vi "Car Wash.vi"() -> ()   [LabVIEW 2021]
uses:
  Controls/Car Wash Indicators.ctl
  Controls/Wash Options.ctl
  Controls/Enum State Machine.ctl
  <vilib>/DAQmx/read.llb/DAQmx Read (Counter U32 1Chan 1Samp).vi
  <vilib>/DAQmx/read.llb/DAQmx Read (Analog 1D Wfm NChan NSamp).vi
  <vilib>/DAQmx/write.llb/DAQmx Write (Analog 1D Wfm NChan NSamp).vi
  <vilib>/DAQmx/miscellaneous.llb/DAQmx Fill In Error Info.vi
  <vilib>/DAQmx/configure/timing.llb/DAQmx Timing (Use Waveform).vi
  <vilib>/measure/NI_MABase.lvlib
panel:
  out "Water Flow Graph":waveform(dbl)[](graph)
  in  "Duty Cycle Control(%)":dbl(slide)=5.0 min=5.0 max=95.0 step=1.0 scale=5.0..95.0 scale format="%.2g"
  out "error out":errorcluster
  in  "error in (no error)":errorcluster
  in  "Data Type":u8
  in  "Wash Options":T1
  in  "Start":bool
  out "Elapsed Time":dbl format="%0.2f"
  in  "stop":bool
  out "Wash Entry":bool
  out "Car Position Slider":u8(slide) max=3 scale=0.0..4.0
  out "CW Indicators":T2
  # "Entry Console"
  # "Car Wash Display"
  # "Car Position Simulation"
  # "Pre-Soak\nH-P Wash\nL-P Wax\nSpot Free Rinse"
  # "Underbody Wash\nBug Remover"
  # "Tire Shine\nAir Dry"
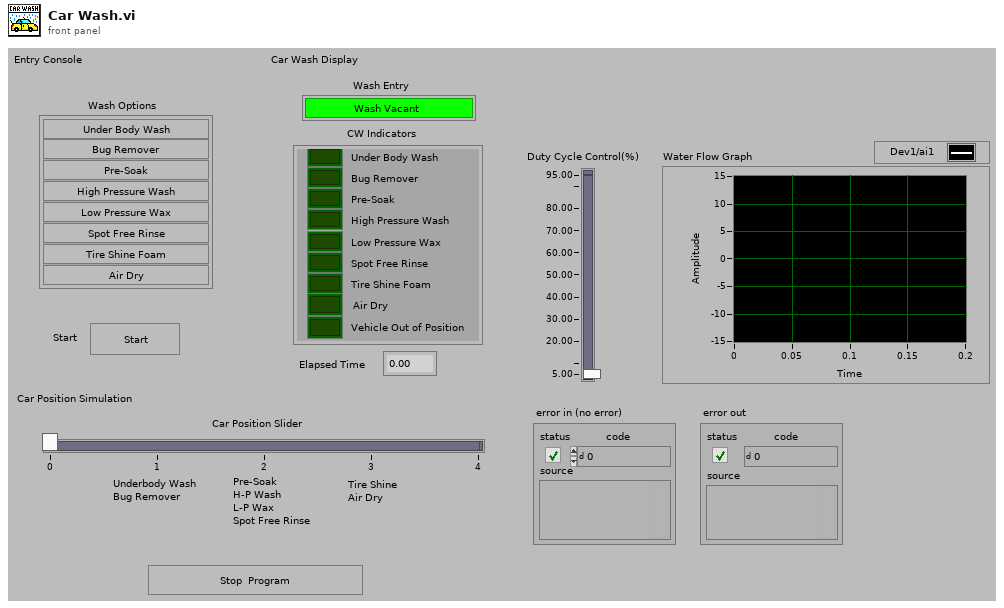
[diagram p1: front panel]
types:
  T1 = typedef "Wash Options.ctl" = cluster{"Underbody Wash":bool, "Bug Remover":bool, "Pre-Soak":bool, "High Pressure Wash":bool, "Low Pressure Wax":bool, "Spot Free Rinse":bool, "Tire Shine Foam":bool, "Air Dry":bool}
  T2 = typedef "Car Wash Indicators.ctl" = cluster{"Vehicle Out of Position":bool, "Under Body Wash":bool, "Bug Remover":bool, "Pre-Soak":bool, "High Pressure Wash":bool, "Low Pressure Wax":bool, "Spot Free Rinse":bool, "Tire Shine Foam":bool, "Air Dry":bool}
  T3 = cluster{"frequency":dbl, "amplitude":dbl, "phase":dbl, "sampling info":cluster{"Fs":dbl, "#s":dbl}}
  T4 = cluster{"maximum value":dbl, "minimum value":dbl, "physical channels":tag}
  T5 = cluster{"minimum value":dbl, "maximum value":dbl, "physical channels":tag, "rate":dbl, "sample mode":i32, "samples per channel":i32}
  T6 = cluster{"initial count":u32, "count direction":i32, "edge":i32, "counter":tag, "CI.CountEdges.Term":tag}
  T7 = typedef "Enum State Machine.ctl" = enum16{"Entry", "Under Body Wash", "Bug Remover", "Pre-Soak", "High Pressure Wash", "Low Pressure Wax", "Spot Free Rinse", "Tire Shine Foam", "Air Dry", "Exit", "Startup", "Wait for Start", "Stop"}
  T8 = cluster{"Car Wash Indicators":T2, "Wash Options":T1}
  T9 = enum8{"Enabled", "Disabled", "Disabled and Grayed Out"}
  T10 = typedef "Car Wash Data.ctl" = cluster{"Car Wash Indicators":T2, "Wash Options":T1}
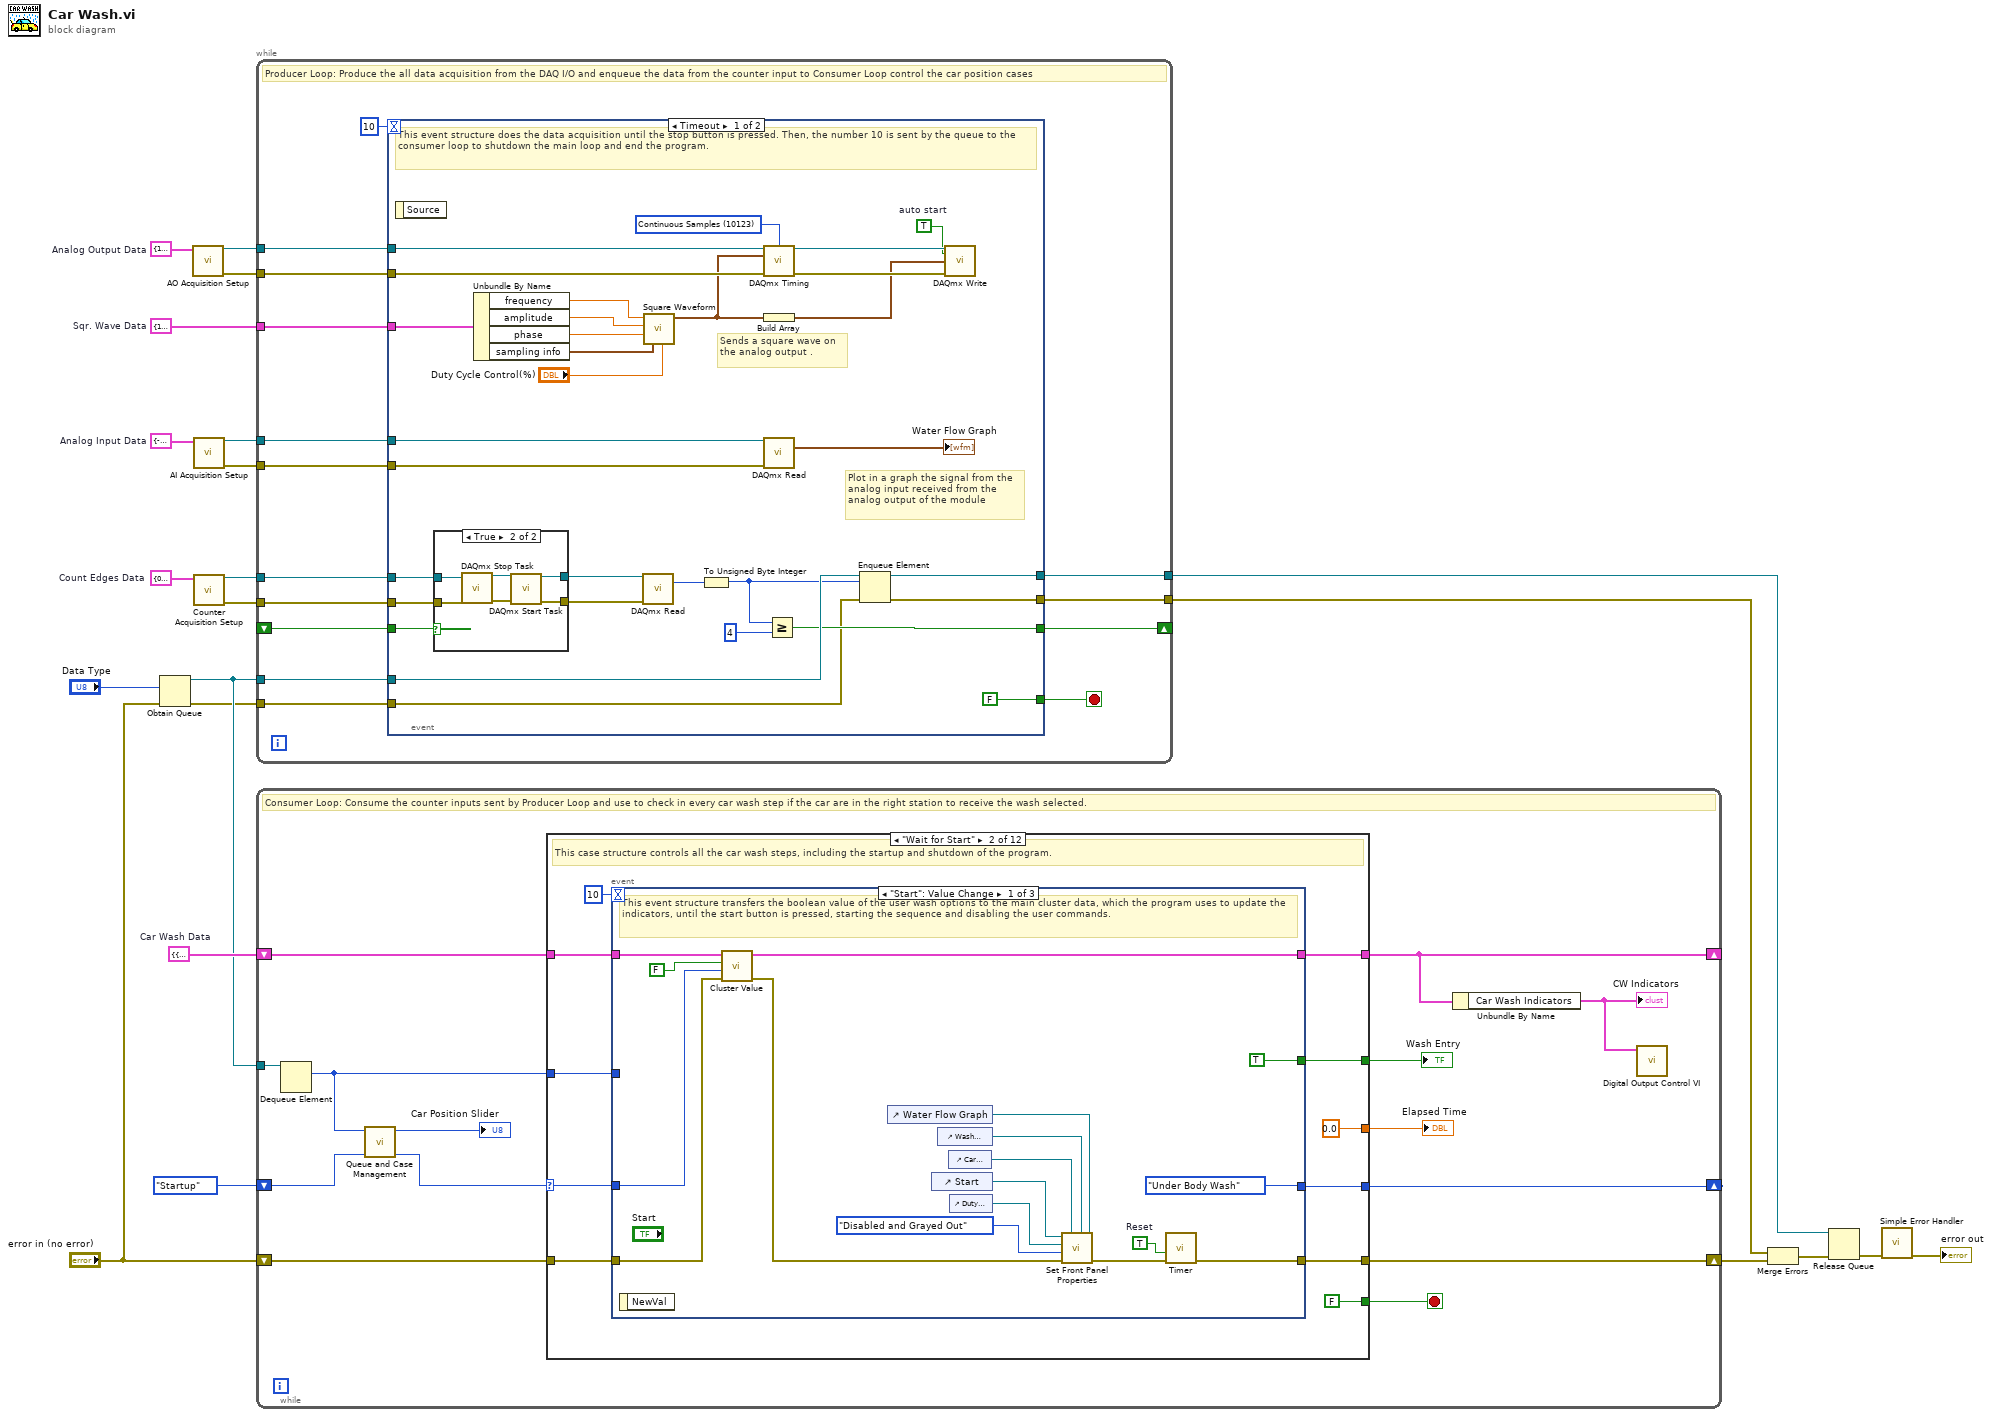
[diagram p0: block diagram]
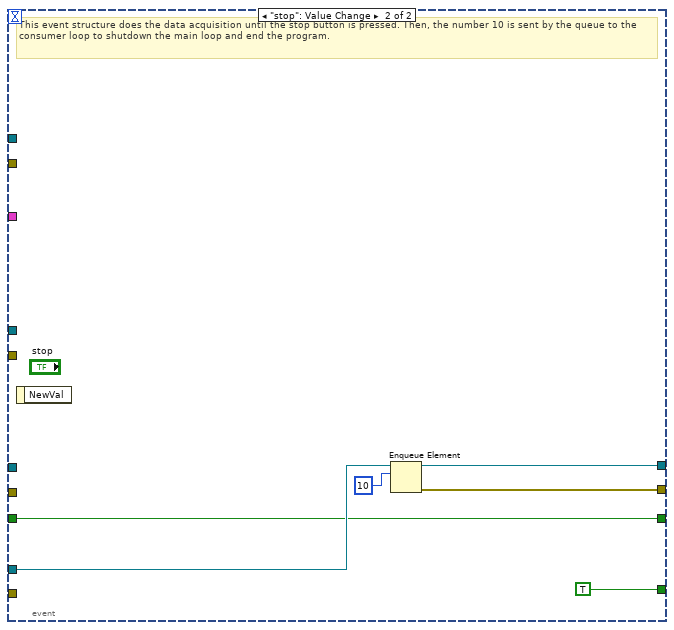
[diagram p3: hidden frame]
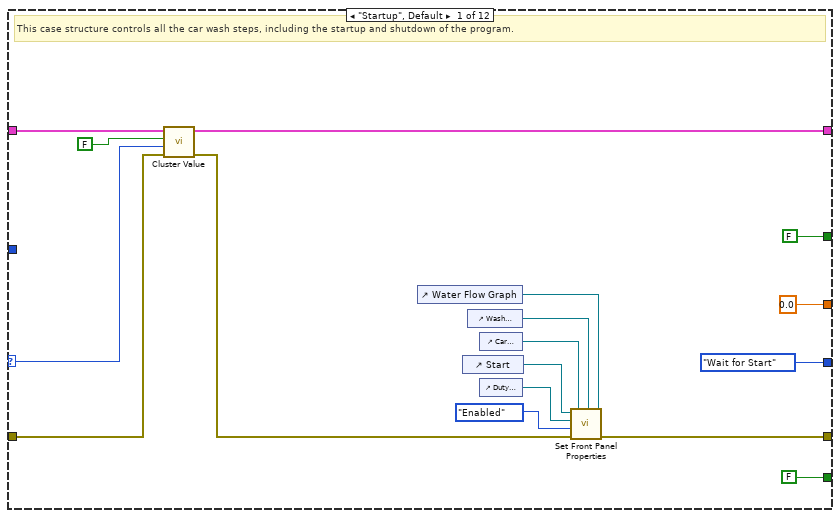
[diagram p4: hidden frame]
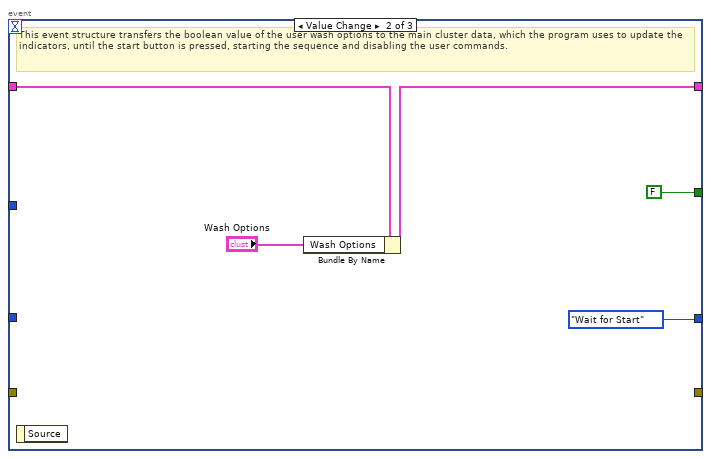
[diagram p5: hidden frame]
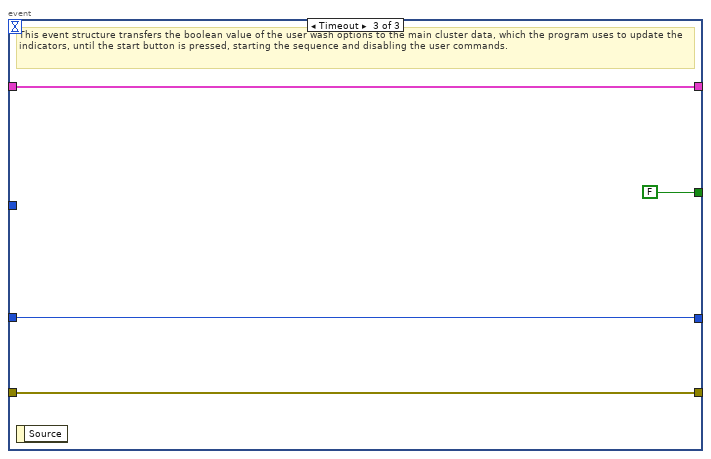
[diagram p6: hidden frame]
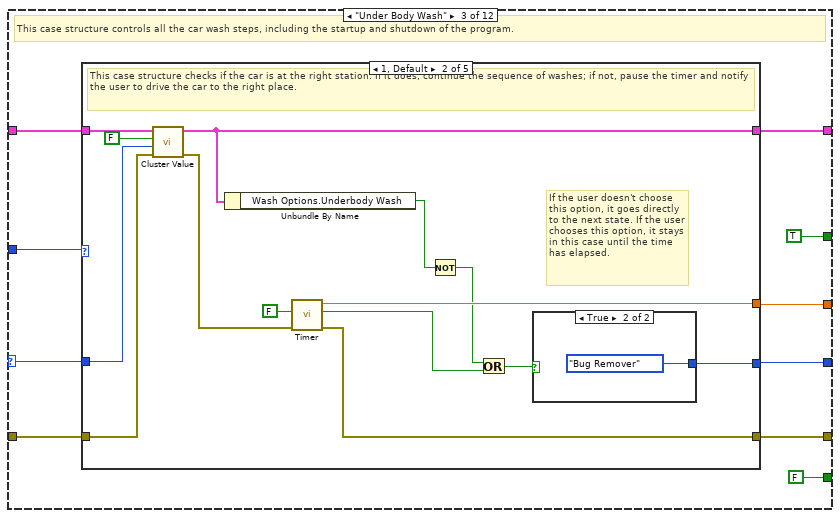
[diagram p7: hidden frame]
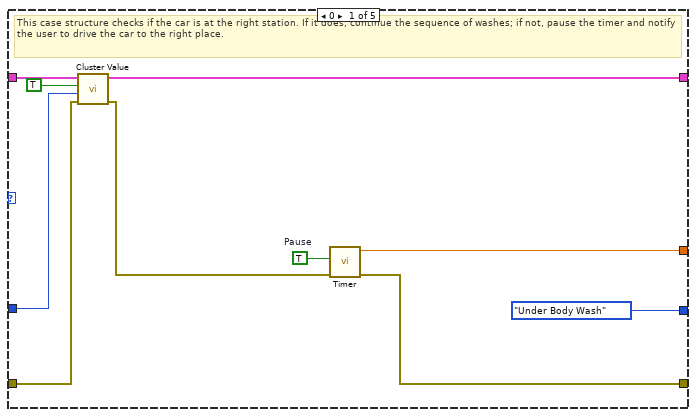
[diagram p8: hidden frame]
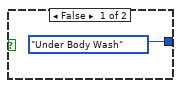
[diagram p9: hidden frame]
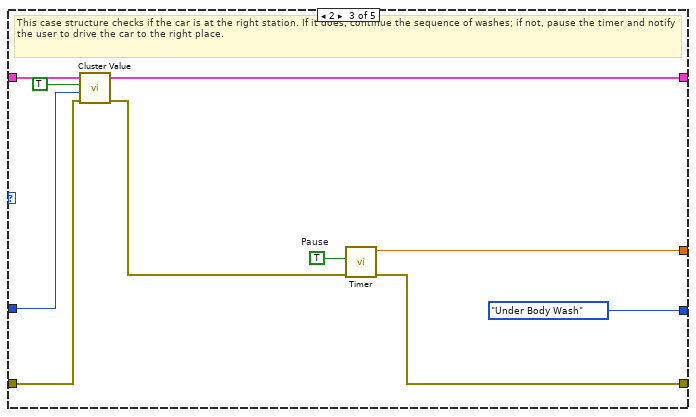
[diagram p10: hidden frame]
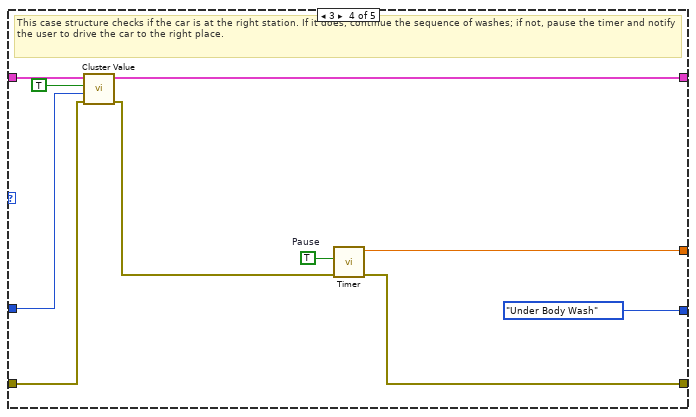
[diagram p11: hidden frame]
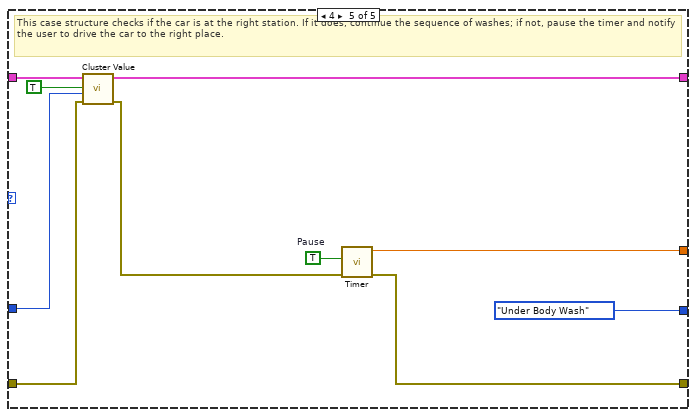
[diagram p12: hidden frame]
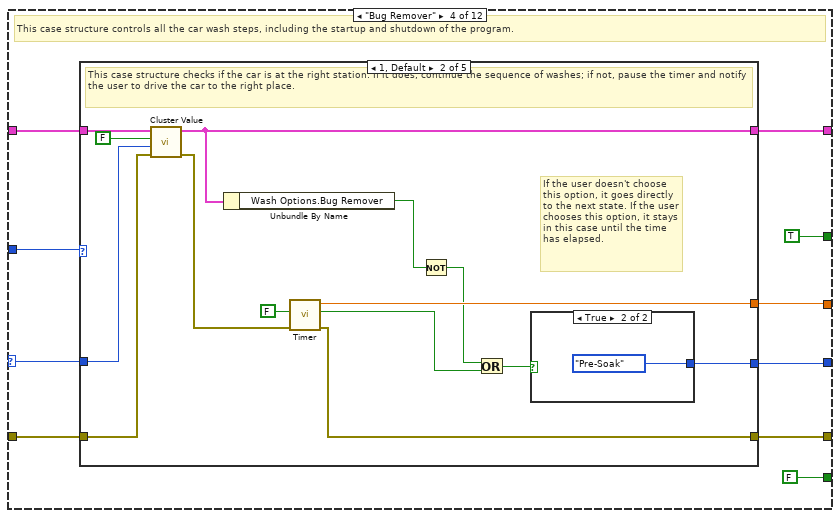
[diagram p13: hidden frame]
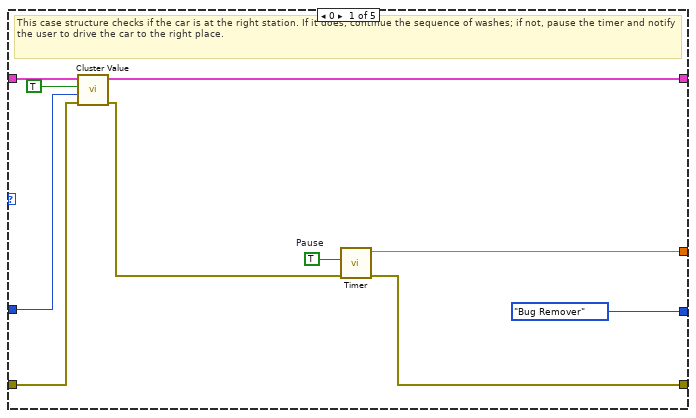
[diagram p14: hidden frame]
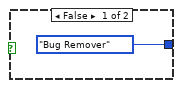
[diagram p15: hidden frame]
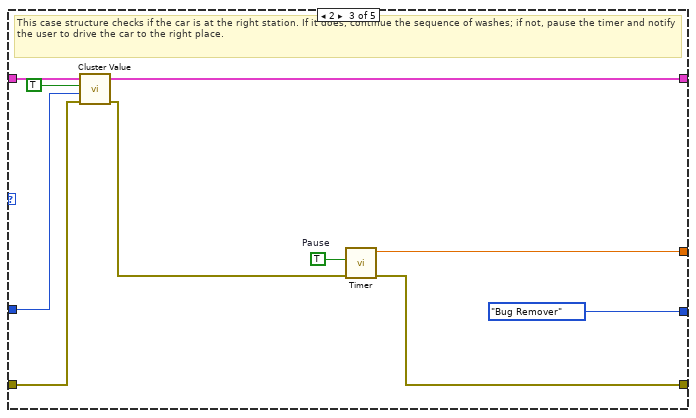
[diagram p16: hidden frame]
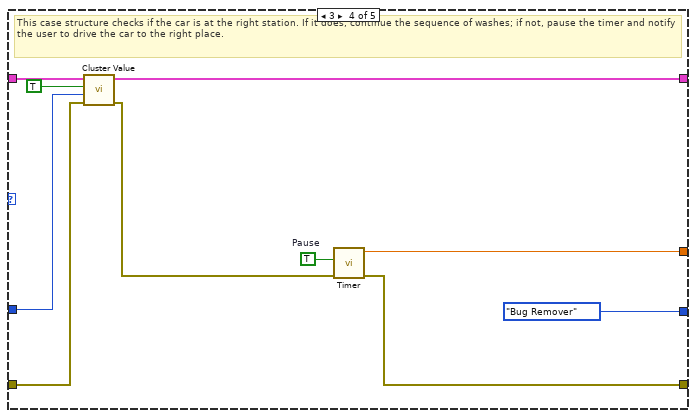
[diagram p17: hidden frame]
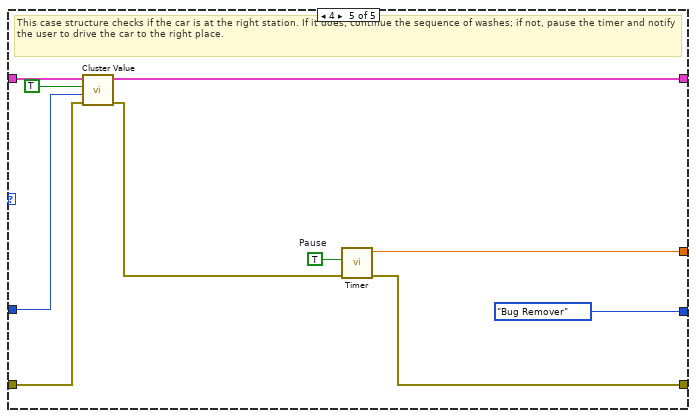
[diagram p18: hidden frame]
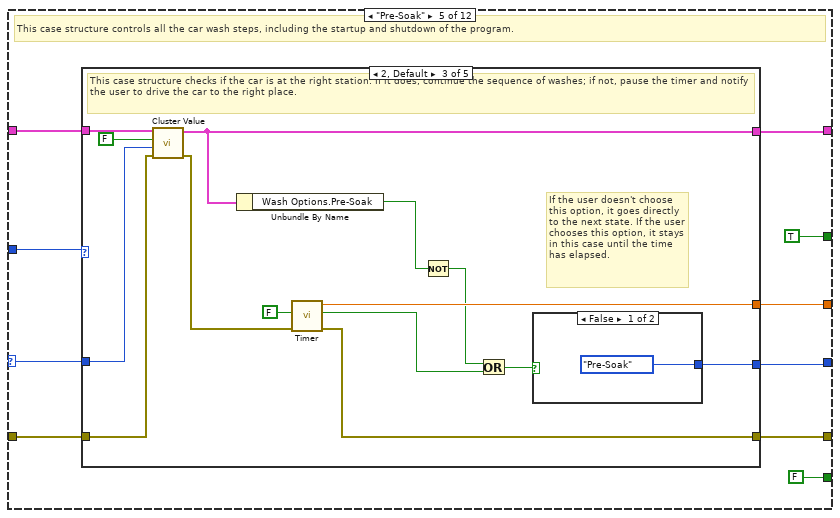
[diagram p19: hidden frame]
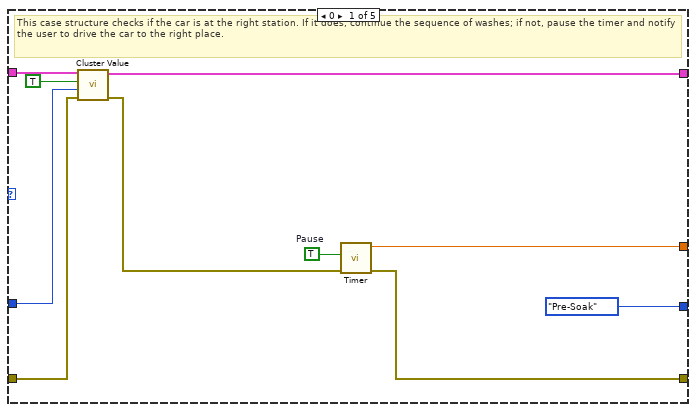
[diagram p20: hidden frame]
diagram:
  w3 = T3 {"frequency"=18.0, "amplitude"=10.0, "phase"=0.0, "sampling info"={"Fs"=1000.0, "#s"=100.0}}  # Sqr. Wave Data
  w5 = T4 {"maximum value"=10.0, "minimum value"=-10.0, "physical channels"="Dev1/ao1"}  # Analog Output Data
  w6 = T5 {"minimum value"=-10.0, "maximum value"=10.0, "physical channels"="Dev1/ai1", "rate"=1800.0, "sample mode"=10123, "samples per channel"=10000}  # Analog Input Data
  w7 = T6 {"initial count"=0, "count direction"=10128, "edge"=10280, "counter"="Dev1/ctr0", "CI.CountEdges.Term"="/Dev1/PFI1"}  # Count Edges Data
  w22 = T8 {"Car Wash Indicators"={"Vehicle Out of Position"=FALSE, "Under Body Wash"=FALSE, "Bug Remover"=FALSE, "Pre-Soak"=FALSE, "High Pressure Wash"=FALSE, "Low Pressure Wax"=FALSE, "Spot Free Rinse"=FALSE, "Tire Shine Foam"=FALSE, "Air Dry"=FALSE}, "Wash Options"={"Underbody Wash"=FALSE, "Bug Remover"=FALSE, "Pre-Soak"=FALSE, "High Pressure Wash"=FALSE, "Low Pressure Wax"=FALSE, "Spot Free Rinse"=FALSE, "Tire Shine Foam"=FALSE, "Air Dry"=FALSE}}  # Car Wash Data
  n1 = Obtain Queue(element data type="Data Type", error in (no error)="error in (no error)") -> (queue out=w20:refnum<queue>, error out=w2:errorcluster)  [unwired: 3 in, 1 out]
  n2 = call "AO Acquisition Setup.vi"("Analog Output Data"=w5) -> ("error out"=w12:errorcluster, "Refnum out"=w16:refnum<k21>)  [unwired: 9 in]
  n3 = call "AI Acquisition Setup.vi"("Analog Input Data"=w6) -> ("error out"=w14:errorcluster, "Refnum out"=w15:refnum<k21>)  [unwired: 9 in]
  n4 = call "Counter Acquisition Setup.vi"("Count Edges Data"=w7) -> ("error out"=w13:errorcluster, "Refnum out"=w17:refnum<k21>)  [unwired: 9 in]
  n5 = while {
    tunnel: w20 -> [w37]
    tunnel: [w36] -> w9
    tunnel: [w35] -> w8
    tunnel: w17 -> [w30]
    tunnel: w16 -> [w34]
    tunnel: w15 -> [w33]
    shift-right: [w32] -> _
    shift-left: _ -> [w31]
    tunnel: w14 -> [w29]
    tunnel: w13 -> [w28]
    tunnel: w12 -> [w27]
    tunnel: w3 -> [w25]
    tunnel: w2 -> [w24]
    stop <- w26 stop-if-true
    # "Producer Loop: Produce the all data acquisition from the DAQ I/O and enqueue the data from the counter input to Consumer Loop control the car position cases"
    n6 = event shown="[0] Timeout" {
      selector: _ -> [_ _]
      dyn-events: _ -> [_ _]
      timeout: 10 -> [_ _]
      tunnel: w37 -> [w68 w80]
      tunnel: [w67 w82] -> w36
      tunnel: [w66 w81] -> w35
      tunnel: w34 -> [w61 _]
      tunnel: w33 -> [w39 _]
      tunnel: [w60 w79] -> w32
      tunnel: w31 -> [w59 w79]
      tunnel: w30 -> [w58 _]
      tunnel: w29 -> [w38 _]
      tunnel: w28 -> [w55 _]
      tunnel: w27 -> [w53 _]
      tunnel: [FALSE TRUE] -> w26
      tunnel: w25 -> [w43 _]
      tunnel: w24 -> [w42 _]
      event Timeout {
        w49 = TRUE  # auto start
        w63 = 10123 items=["Finite Samples"=10178, "Continuous Samples"=10123, "Hardware Timed Single Point"=12522] ("sample mode")
        # "Plot in a graph the signal from the analog input received from the analog output of the module"
        # "Sends a square wave on the analog output ."
        # "This event structure does the data acquisition until the stop button is pressed. Then, the number 10 is sent by the queue to the consumer loop to shutdown the main loop and end the program."
        n7 = event-data() -> ()  [unwired: 1 in, 1 out]
        n8 = case shown="True" w59 {
          tunnel: w58 -> [w70 w76]
          tunnel: [w70 w74] -> w57
          tunnel: w55 -> [w69 w73]
          tunnel: [w69 w71] -> w54
          frame False {
          }
          frame True {
            n9 = call <vilib>:"DAQmx Stop Task.vi"("task/channels in"=w76, "error in"=w73) -> ("task out"=w75:refnum<k21>, "error out"=w72:errorcluster)  [unwired: 12 in]
            n10 = call <vilib>:"DAQmx Start Task.vi"("task/channels in"=w75, "error in"=w72) -> ("task out"=w74:refnum<k21>, "error out"=w71:errorcluster)  [unwired: 12 in]
          }
        }
        n11 = Unbundle By Name(w43) -> ("frequency"=w48:dbl, "amplitude"=w47:dbl, "phase"=w46:dbl, "sampling info"=w45:cluster{"Fs":dbl, "#s":dbl})
        n12 = call-poly <vilib>:"DAQmx Read.vi"("task/channels in"=w57, "error in"=w54) -> ("data"=w62:u32)  [unwired: 11 in, 2 out]
        n13 = call <vilib>:"Square Waveform.vi"("duty cycle (%)"="Duty Cycle Control(%)", "sampling info"=w45, "phase"=w46, "amplitude"=w47, "frequency"=w48) -> ("signal out"=w41:waveform(dbl))  [unwired: 5 in, 1 out]
        n14 = To Unsigned Byte Integer(number=w62) -> (unsigned 8bit integer=w56:u8)
        n15 = call-poly <vilib>:"DAQmx Timing.vi"("task/channels in"=w61, "sample mode"=w63, "waveform"=w41, "error in"=w53) -> ("task out"=w64:refnum<k21>, "error out"=w52:errorcluster)  [unwired: 10 in]
        n16 = Build Array(w41) -> (w51:waveform(dbl)[])
        n17 = call-poly <vilib>:"DAQmx Read.vi"("task/channels in"=w39, "error in"=w38) -> ("data"=→"Water Flow Graph":waveform(dbl)[])  [unwired: 11 in, 2 out]
        n18 = Greater Or Equal?(x=w56, y=u8 4) -> (x >= y?=w60:bool)
        n19 = Enqueue Element(queue=w68, element=w56, error in (no error)=w42) -> (queue out=w67:refnum<queue>, error out=w66:errorcluster)  [unwired: 1 in, 1 out]
        n20 = call-poly <vilib>:"DAQmx Write.vi"("task/channels in"=w64, "auto start"=w49, "data"=w51, "error in"=w52) -> ()  [unwired: 9 in, 3 out]
      }
      event "stop": Value Change {
        # "This event structure does the data acquisition until the stop button is pressed. Then, the number 10 is sent by the queue to the consumer loop to shutdown the main loop and end the program."
        n21 = event-data() -> ()  [unwired: 1 in, 1 out]
        n22 = Enqueue Element(queue=w80, element=u8 10) -> (queue out=w82:refnum<queue>, error out=w81:errorcluster)  [unwired: 2 in, 1 out]
      }
    }
  }
  n23 = while {
    shift-right: [w87] -> _
    shift-left: Enum_State_Machine."Startup" ("Enum") -> [w83]
    shift-right: [w93] -> _
    shift-left: w22 -> [w94]
    tunnel: w20 -> [w91]
    shift-right: [w89] -> w18
    shift-left: "error in (no error)" -> [w88]
    stop <- w92 stop-if-true
    # "Consumer Loop: Consume the counter inputs sent by Producer Loop and use to check in every car wash step if the car are in the right station to receive the wash selected."
    n24 = Dequeue Element(queue=w91) -> (element=w86:u8)  [unwired: 2 in, 3 out]
    n25 = call "Queue and Case Management.vi"("States input"=w83, "Queue element"=w86) -> ("States output"=w84:T7, "Slider output"=→"Car Position Slider":u8)  [unwired: 8 in]
    n26 = case shown="\"Wait for Start\"" w84 {
      selector: w84 -> [w100 w120 w157 w220 w289 w354 w416 w481 w547 w613 w681 w731]
      tunnel: [Enum_State_Machine."Wait for Start" w124 w158 w219 w285 w351 w418 w479 w545 w610 w680 w731] -> w87
      tunnel: w94 -> [w103 w123 w155 w224 w287 w356 w414 w483 w549 w616 w683 w736]
      tunnel: [w102 w122 w159 w221 w284 w355 w413 w484 w550 w615 w682 w735] -> w93
      tunnel: [FALSE ("Wash Entry") w121 TRUE ("Wash Entry") TRUE ("Wash Entry") TRUE ("Wash Entry") TRUE ("Wash Entry") TRUE ("Wash Entry") TRUE ("Wash Entry") TRUE ("Wash Entry") TRUE ("Wash Entry") TRUE ("Wash Entry") FALSE ("Wash Entry")] -> w96
      tunnel: [0.0 ("Elapsed Time (s)") 0.0 ("Elapsed Time (s)") w154 w218 w286 w350 w417 w478 w544 w611 0.0 ("Elapsed Time (s)") 0.0 ("Elapsed Time (s)")] -> w95
      tunnel: w86 -> [_ w118 w156 w223 w288 w353 w415 w482 w548 w614 w679 _]
      tunnel: [FALSE FALSE FALSE FALSE FALSE FALSE FALSE FALSE FALSE FALSE FALSE TRUE] -> w92
      tunnel: [w109 w115 w153 w222 w290 w352 w419 w480 w546 w612 w676 w730] -> w89
      tunnel: w88 -> [w99 w116 w152 w217 w283 w349 w412 w477 w543 w609 w675 w726]
      frame "Startup", Default {
        # "This case structure controls all the car wash steps, including the startup and shutdown of the program."
        n27 = call "Cluster Value.vi"("error in (no error)"=w99, "Enum Input"=w100, "Vehicle Out of Position"=FALSE, "Data Car Wash"=w103) -> ("error out"=w98:errorcluster, "Data Car Wash Output"=w102:T10)  [unwired: 6 in]
        n28 = control-ref of="Water Flow Graph"() -> (w97:refnum<vi>)
        n29 = control-ref of="Start"() -> (w106:refnum<vi>)
        n30 = control-ref of="Wash Options"() -> (w108:refnum<vi>)
        n31 = control-ref of="Car Position Slider"() -> (w107:refnum<vi>)
        n32 = control-ref of="Duty Cycle Control(%)"() -> (w105:refnum<vi>)
        n33 = call "Set Front Panel Properties.vi"("Water Flow Graph Refnum"=w97, "Wash Op Refnum"=w108, "Car Slider Refnum"=w107, "error in (no error)"=w98, "Control"=T9."Enabled", "DtCy Slider Refnum"=w105, "Start Refnum"=w106) -> ("error out"=w109:errorcluster)  [unwired: 4 in]
      }
      frame "Wait for Start" {
        # "This case structure controls all the car wash steps, including the startup and shutdown of the program."
        n34 = event shown="[0] \"Start\": Value Change" {
          selector: _ -> [_ _ _]
          dyn-events: _ -> [_ _ _]
          timeout: 10 -> [_ _ _]
          tunnel: [Enum_State_Machine."Under Body Wash" Enum_State_Machine."Wait for Start" w149] -> w124
          tunnel: w123 -> [w141 w146 w150]
          tunnel: [w140 w144 w150] -> w122
          tunnel: [TRUE ("Wash Entry") FALSE ("Wash Entry") FALSE ("Wash Entry")] -> w121
          tunnel: w120 -> [w136 _ w149]
          tunnel: w118 -> [_ _ _]
          tunnel: w116 -> [w129 _ w148]
          tunnel: [w127 _ w148] -> w115
          event "Start": Value Change {
            w135 = TRUE  # Reset
            # "This event structure transfers the boolean value of the user wash options to the main cluster data, which the program uses to update the indicators, until the start button is pressed, starting the sequence and disabling the user commands."
            n35 = event-data() -> ()  [unwired: 1 in, 1 out]
            n36 = call "Cluster Value.vi"("error in (no error)"=w129, "Enum Input"=w136, "Vehicle Out of Position"=FALSE, "Data Car Wash"=w141) -> ("error out"=w126:errorcluster, "Data Car Wash Output"=w140:T10)  [unwired: 6 in]
            n37 = control-ref of="Water Flow Graph"() -> (w125:refnum<vi>)
            n38 = control-ref of="Start"() -> (w130:refnum<vi>)
            n39 = control-ref of="Wash Options"() -> (w134:refnum<vi>)
            n40 = control-ref of="Car Position Slider"() -> (w133:refnum<vi>)
            n41 = control-ref of="Duty Cycle Control(%)"() -> (w131:refnum<vi>)
            n42 = call "Set Front Panel Properties.vi"("Water Flow Graph Refnum"=w125, "Wash Op Refnum"=w134, "Car Slider Refnum"=w133, "error in (no error)"=w126, "Control"=T9."Disabled and Grayed Out", "DtCy Slider Refnum"=w131, "Start Refnum"=w130) -> ("error out"=w128:errorcluster)  [unwired: 4 in]
            n43 = call "Timer.vi"("error in (no error)"=w128, "Reset"=w135) -> ("error out"=w127:errorcluster)  [unwired: 6 in, 2 out]
          }
          event Value Change {
            # "This event structure transfers the boolean value of the user wash options to the main cluster data, which the program uses to update the indicators, until the start button is pressed, starting the sequence and disabling the user commands."
            n44 = event-data() -> ()  [unwired: 1 in, 1 out]
            n45 = Bundle By Name(cluster=w146, "Wash Options"="Wash Options") -> (w144:T10)
          }
          event Timeout {
            # "This event structure transfers the boolean value of the user wash options to the main cluster data, which the program uses to update the indicators, until the start button is pressed, starting the sequence and disabling the user commands."
            n46 = event-data() -> ()  [unwired: 1 in, 1 out]
          }
        }
      }
      frame "Under Body Wash" {
        # "This case structure controls all the car wash steps, including the startup and shutdown of the program."
        n47 = case shown="1, Default" w156 {
          tunnel: [Enum_State_Machine."Under Body Wash" w182 Enum_State_Machine."Under Body Wash" Enum_State_Machine."Under Body Wash" Enum_State_Machine."Under Body Wash"] -> w158
          tunnel: w155 -> [w169 w184 w195 w206 w215]
          tunnel: [w168 w183 w194 w205 w216] -> w159
          tunnel: w157 -> [w164 w176 w190 w200 w210]
          tunnel: [w166 w180 w193 w203 w213] -> w154
          tunnel: [w162 w174 w188 w198 w208] -> w153
          tunnel: w152 -> [w161 w171 w187 w197 w207]
          frame 0 {
            w167 = TRUE  # Pause
            # "This case structure checks if the car is at the right station. If it does, continue the sequence of washes; if not, pause the timer and notify the user to drive the car to the right place."
            n48 = call "Cluster Value.vi"("error in (no error)"=w161, "Enum Input"=w164, "Vehicle Out of Position"=TRUE, "Data Car Wash"=w169) -> ("error out"=w163:errorcluster, "Data Car Wash Output"=w168:T10)  [unwired: 6 in]
            n49 = call "Timer.vi"("error in (no error)"=w163, "Pause"=w167) -> ("error out"=w162:errorcluster, "Elapsed Time"=w166:dbl)  [unwired: 6 in, 1 out]
          }
          frame 1, Default {
            # "If the user doesn't choose this option, it goes directly to the next state. If the user chooses this option, it stays in this case until the time has elapsed."
            # "This case structure checks if the car is at the right station. If it does, continue the sequence of washes; if not, pause the timer and notify the user to drive the car to the right place."
            n50 = call "Cluster Value.vi"("error in (no error)"=w171, "Enum Input"=w176, "Vehicle Out of Position"=FALSE, "Data Car Wash"=w184) -> ("error out"=w175:errorcluster, "Data Car Wash Output"=w183:T10)  [unwired: 6 in]
            n51 = Unbundle By Name(w183) -> ("Wash Options.Underbody Wash"=w178:bool)
            n52 = call "Timer.vi"("error in (no error)"=w175, "Pause"=FALSE) -> ("error out"=w174:errorcluster, "Time Has Elapsed?"=w172:bool, "Elapsed Time"=w180:dbl)  [unwired: 6 in]
            n53 = Not(x=w178) -> (.not. x?=w177:bool)
            n54 = Or(x=w177, y=w172) -> (x .or. y?=w179:bool)
            n55 = case shown="True" w179 {
              tunnel: [Enum_State_Machine."Under Body Wash" ("Enum") Enum_State_Machine."Bug Remover" ("Enum")] -> w182
              frame False {
              }
              frame True {
              }
            }
          }
          frame 2 {
            w192 = TRUE  # Pause
            # "This case structure checks if the car is at the right station. If it does, continue the sequence of washes; if not, pause the timer and notify the user to drive the car to the right place."
            n56 = call "Cluster Value.vi"("error in (no error)"=w187, "Enum Input"=w190, "Vehicle Out of Position"=TRUE, "Data Car Wash"=w195) -> ("error out"=w189:errorcluster, "Data Car Wash Output"=w194:T10)  [unwired: 6 in]
            n57 = call "Timer.vi"("error in (no error)"=w189, "Pause"=w192) -> ("error out"=w188:errorcluster, "Elapsed Time"=w193:dbl)  [unwired: 6 in, 1 out]
          }
          frame 3 {
            w204 = TRUE  # Pause
            # "This case structure checks if the car is at the right station. If it does, continue the sequence of washes; if not, pause the timer and notify the user to drive the car to the right place."
            n58 = call "Cluster Value.vi"("error in (no error)"=w197, "Enum Input"=w200, "Vehicle Out of Position"=TRUE, "Data Car Wash"=w206) -> ("error out"=w199:errorcluster, "Data Car Wash Output"=w205:T10)  [unwired: 6 in]
            n59 = call "Timer.vi"("error in (no error)"=w199, "Pause"=w204) -> ("error out"=w198:errorcluster, "Elapsed Time"=w203:dbl)  [unwired: 6 in, 1 out]
          }
          frame 4 {
            w214 = TRUE  # Pause
            # "This case structure checks if the car is at the right station. If it does, continue the sequence of washes; if not, pause the timer and notify the user to drive the car to the right place."
            n60 = call "Cluster Value.vi"("error in (no error)"=w207, "Enum Input"=w210, "Vehicle Out of Position"=TRUE, "Data Car Wash"=w215) -> ("error out"=w209:errorcluster, "Data Car Wash Output"=w216:T10)  [unwired: 6 in]
            n61 = call "Timer.vi"("error in (no error)"=w209, "Pause"=w214) -> ("error out"=w208:errorcluster, "Elapsed Time"=w213:dbl)  [unwired: 6 in, 1 out]
          }
        }
      }
      frame "Bug Remover" {
        # "This case structure controls all the car wash steps, including the startup and shutdown of the program."
        n62 = case shown="1, Default" w223 {
          tunnel: [Enum_State_Machine."Bug Remover" w249 Enum_State_Machine."Bug Remover" Enum_State_Machine."Bug Remover" Enum_State_Machine."Bug Remover"] -> w219
          tunnel: [w235 w250 w261 w272 w282] -> w221
          tunnel: [w233 w247 w260 w270 w280] -> w218
          tunnel: w224 -> [w232 w243 w258 w268 w278]
          tunnel: [w228 w239 w254 w264 w274] -> w222
          tunnel: w220 -> [w230 w241 w256 w266 w276]
          tunnel: w217 -> [w227 w237 w253 w263 w273]
          frame 0 {
            w234 = TRUE  # Pause
            # "This case structure checks if the car is at the right station. If it does, continue the sequence of washes; if not, pause the timer and notify the user to drive the car to the right place."
            n63 = call "Cluster Value.vi"("error in (no error)"=w227, "Enum Input"=w230, "Vehicle Out of Position"=TRUE, "Data Car Wash"=w232) -> ("error out"=w229:errorcluster, "Data Car Wash Output"=w235:T10)  [unwired: 6 in]
            n64 = call "Timer.vi"("error in (no error)"=w229, "Pause"=w234) -> ("error out"=w228:errorcluster, "Elapsed Time"=w233:dbl)  [unwired: 6 in, 1 out]
          }
          frame 1, Default {
            # "If the user doesn't choose this option, it goes directly to the next state. If the user chooses this option, it stays in this case until the time has elapsed."
            # "This case structure checks if the car is at the right station. If it does, continue the sequence of washes; if not, pause the timer and notify the user to drive the car to the right place."
            n65 = call "Cluster Value.vi"("error in (no error)"=w237, "Enum Input"=w241, "Vehicle Out of Position"=FALSE, "Data Car Wash"=w243) -> ("error out"=w240:errorcluster, "Data Car Wash Output"=w250:T10)  [unwired: 6 in]
            n66 = Unbundle By Name(w250) -> ("Wash Options.Bug Remover"=w245:bool)
            n67 = call "Timer.vi"("error in (no error)"=w240, "Pause"=FALSE) -> ("error out"=w239:errorcluster, "Time Has Elapsed?"=w238:bool, "Elapsed Time"=w247:dbl)  [unwired: 6 in]
            n68 = Not(x=w245) -> (.not. x?=w244:bool)
            n69 = Or(x=w244, y=w238) -> (x .or. y?=w246:bool)
            n70 = case shown="True" w246 {
              tunnel: [Enum_State_Machine."Bug Remover" ("Enum") Enum_State_Machine."Pre-Soak" ("Enum")] -> w249
              frame False {
              }
              frame True {
              }
            }
          }
          frame 2 {
            w259 = TRUE  # Pause
            # "This case structure checks if the car is at the right station. If it does, continue the sequence of washes; if not, pause the timer and notify the user to drive the car to the right place."
            n71 = call "Cluster Value.vi"("error in (no error)"=w253, "Enum Input"=w256, "Vehicle Out of Position"=TRUE, "Data Car Wash"=w258) -> ("error out"=w255:errorcluster, "Data Car Wash Output"=w261:T10)  [unwired: 6 in]
            n72 = call "Timer.vi"("error in (no error)"=w255, "Pause"=w259) -> ("error out"=w254:errorcluster, "Elapsed Time"=w260:dbl)  [unwired: 6 in, 1 out]
          }
          frame 3 {
            w271 = TRUE  # Pause
            # "This case structure checks if the car is at the right station. If it does, continue the sequence of washes; if not, pause the timer and notify the user to drive the car to the right place."
            n73 = call "Cluster Value.vi"("error in (no error)"=w263, "Enum Input"=w266, "Vehicle Out of Position"=TRUE, "Data Car Wash"=w268) -> ("error out"=w265:errorcluster, "Data Car Wash Output"=w272:T10)  [unwired: 6 in]
            n74 = call "Timer.vi"("error in (no error)"=w265, "Pause"=w271) -> ("error out"=w264:errorcluster, "Elapsed Time"=w270:dbl)  [unwired: 6 in, 1 out]
          }
          frame 4 {
            w281 = TRUE  # Pause
            # "This case structure checks if the car is at the right station. If it does, continue the sequence of washes; if not, pause the timer and notify the user to drive the car to the right place."
            n75 = call "Cluster Value.vi"("error in (no error)"=w273, "Enum Input"=w276, "Vehicle Out of Position"=TRUE, "Data Car Wash"=w278) -> ("error out"=w275:errorcluster, "Data Car Wash Output"=w282:T10)  [unwired: 6 in]
            n76 = call "Timer.vi"("error in (no error)"=w275, "Pause"=w281) -> ("error out"=w274:errorcluster, "Elapsed Time"=w280:dbl)  [unwired: 6 in, 1 out]
          }
        }
      }
      frame "Pre-Soak" {
        # "This case structure controls all the car wash steps, including the startup and shutdown of the program."
        n77 = case shown="2, Default" w288 {
          tunnel: [Enum_State_Machine."Pre-Soak" Enum_State_Machine."Pre-Soak" w325 Enum_State_Machine."Pre-Soak" Enum_State_Machine."Pre-Soak"] -> w285
          tunnel: [w301 w311 w326 w338 w348] -> w284
          tunnel: [w299 w310 w323 w336 w346] -> w286
          tunnel: [w294 w304 w315 w330 w340] -> w290
          tunnel: w289 -> [w296 w306 w317 w332 w342]
          tunnel: w287 -> [w298 w308 w319 w334 w344]
          tunnel: w283 -> [w293 w303 w313 w329 w339]
          frame 0 {
            w300 = TRUE  # Pause
            # "This case structure checks if the car is at the right station. If it does, continue the sequence of washes; if not, pause the timer and notify the user to drive the car to the right place."
            n78 = call "Cluster Value.vi"("error in (no error)"=w293, "Enum Input"=w296, "Vehicle Out of Position"=TRUE, "Data Car Wash"=w298) -> ("error out"=w295:errorcluster, "Data Car Wash Output"=w301:T10)  [unwired: 6 in]
            n79 = call "Timer.vi"("error in (no error)"=w295, "Pause"=w300) -> ("error out"=w294:errorcluster, "Elapsed Time"=w299:dbl)  [unwired: 6 in, 1 out]
          }
          frame 1 {
            w309 = TRUE  # Pause
            # "This case structure checks if the car is at the right station. If it does, continue the sequence of washes; if not, pause the timer and notify the user to drive the car to the right place."
            n80 = call "Cluster Value.vi"("error in (no error)"=w303, "Enum Input"=w306, "Vehicle Out of Position"=TRUE, "Data Car Wash"=w308) -> ("error out"=w305:errorcluster, "Data Car Wash Output"=w311:T10)  [unwired: 6 in]
            n81 = call "Timer.vi"("error in (no error)"=w305, "Pause"=w309) -> ("error out"=w304:errorcluster, "Elapsed Time"=w310:dbl)  [unwired: 6 in, 1 out]
          }
          frame 2, Default {
            # "If the user doesn't choose this option, it goes directly to the next state. If the user chooses this option, it stays in this case until the time has elapsed."
            # "This case structure checks if the car is at the right station. If it does, continue the sequence of washes; if not, pause the timer and notify the user to drive the car to the right place."
            n82 = call "Cluster Value.vi"("error in (no error)"=w313, "Enum Input"=w317, "Vehicle Out of Position"=FALSE, "Data Car Wash"=w319) -> ("error out"=w316:errorcluster, "Data Car Wash Output"=w326:T10)  [unwired: 6 in]
            n83 = Unbundle By Name(w326) -> ("Wash Options.Pre-Soak"=w321:bool)
            n84 = call "Timer.vi"("error in (no error)"=w316, "Pause"=FALSE) -> ("error out"=w315:errorcluster, "Time Has Elapsed?"=w314:bool, "Elapsed Time"=w323:dbl)  [unwired: 6 in]
            n85 = Not(x=w321) -> (.not. x?=w320:bool)
            n86 = Or(x=w320, y=w314) -> (x .or. y?=w322:bool)
            n87 = case shown="False" w322 {
              tunnel: [Enum_State_Machine."Pre-Soak" ("Enum") Enum_State_Machine."High Pressure Wash" ("Enum")] -> w325
              frame False {
              }
              frame True {
              }
            }
          }
          frame 3 {
            w337 = TRUE  # Pause
            # "This case structure checks if the car is at the right station. If it does, continue the sequence of washes; if not, pause the timer and notify the user to drive the car to the right place."
            n88 = call "Cluster Value.vi"("error in (no error)"=w329, "Enum Input"=w332, "Vehicle Out of Position"=TRUE, "Data Car Wash"=w334) -> ("error out"=w331:errorcluster, "Data Car Wash Output"=w338:T10)  [unwired: 6 in]
            n89 = call "Timer.vi"("error in (no error)"=w331, "Pause"=w337) -> ("error out"=w330:errorcluster, "Elapsed Time"=w336:dbl)  [unwired: 6 in, 1 out]
          }
          frame 4 {
            w347 = TRUE  # Pause
            # "This case structure checks if the car is at the right station. If it does, continue the sequence of washes; if not, pause the timer and notify the user to drive the car to the right place."
            n90 = call "Cluster Value.vi"("error in (no error)"=w339, "Enum Input"=w342, "Vehicle Out of Position"=TRUE, "Data Car Wash"=w344) -> ("error out"=w341:errorcluster, "Data Car Wash Output"=w348:T10)  [unwired: 6 in]
            n91 = call "Timer.vi"("error in (no error)"=w341, "Pause"=w347) -> ("error out"=w340:errorcluster, "Elapsed Time"=w346:dbl)  [unwired: 6 in, 1 out]
          }
        }
      }
      frame "High Pressure Wash" {
        # "This case structure controls all the car wash steps, including the startup and shutdown of the program."
        n92 = case shown="2, Default" w353 {
          tunnel: [Enum_State_Machine."High Pressure Wash" Enum_State_Machine."High Pressure Wash" w387 Enum_State_Machine."High Pressure Wash" Enum_State_Machine."High Pressure Wash"] -> w351
          tunnel: w356 -> [w367 w377 w389 w401 w410]
          tunnel: [w366 w376 w388 w400 w411] -> w355
          tunnel: w354 -> [w362 w372 w383 w395 w405]
          tunnel: [w364 w375 w385 w398 w408] -> w350
          tunnel: [w360 w370 w381 w393 w403] -> w352
          tunnel: w349 -> [w359 w369 w380 w392 w402]
          frame 0 {
            w365 = TRUE  # Pause
            # "This case structure checks if the car is at the right station. If it does, continue the sequence of washes; if not, pause the timer and notify the user to drive the car to the right place."
            n93 = call "Cluster Value.vi"("error in (no error)"=w359, "Enum Input"=w362, "Vehicle Out of Position"=TRUE, "Data Car Wash"=w367) -> ("error out"=w361:errorcluster, "Data Car Wash Output"=w366:T10)  [unwired: 6 in]
            n94 = call "Timer.vi"("error in (no error)"=w361, "Pause"=w365) -> ("error out"=w360:errorcluster, "Elapsed Time"=w364:dbl)  [unwired: 6 in, 1 out]
          }
          frame 1 {
            w374 = TRUE  # Pause
            # "This case structure checks if the car is at the right station. If it does, continue the sequence of washes; if not, pause the timer and notify the user to drive the car to the right place."
            n95 = call "Cluster Value.vi"("error in (no error)"=w369, "Enum Input"=w372, "Vehicle Out of Position"=TRUE, "Data Car Wash"=w377) -> ("error out"=w371:errorcluster, "Data Car Wash Output"=w376:T10)  [unwired: 6 in]
            n96 = call "Timer.vi"("error in (no error)"=w371, "Pause"=w374) -> ("error out"=w370:errorcluster, "Elapsed Time"=w375:dbl)  [unwired: 6 in, 1 out]
          }
          frame 2, Default {
            # "The high pressure wash is the default option. It will\nexecutate even if the user doesn't choose this option.\nThe next state starts when the time has elapsed."
            # "This case structure checks if the car is at the right station. If it does, continue the sequence of washes; if not, pause the timer and notify the user to drive the car to the right place."
            n97 = call "Cluster Value.vi"("error in (no error)"=w380, "Enum Input"=w383, "Vehicle Out of Position"=FALSE, "Data Car Wash"=w389) -> ("error out"=w382:errorcluster, "Data Car Wash Output"=w388:T10)  [unwired: 6 in]
            n98 = call "Timer.vi"("error in (no error)"=w382, "Pause"=FALSE) -> ("error out"=w381:errorcluster, "Time Has Elapsed?"=w379:bool, "Elapsed Time"=w385:dbl)  [unwired: 6 in]
            n99 = case shown="True" w379 {
              tunnel: [Enum_State_Machine."High Pressure Wash" ("Enum") Enum_State_Machine."Low Pressure Wax" ("Enum")] -> w387
              frame False {
              }
              frame True {
              }
            }
          }
          frame 3 {
            w399 = TRUE  # Pause
            # "This case structure checks if the car is at the right station. If it does, continue the sequence of washes; if not, pause the timer and notify the user to drive the car to the right place."
            n100 = call "Cluster Value.vi"("error in (no error)"=w392, "Enum Input"=w395, "Vehicle Out of Position"=TRUE, "Data Car Wash"=w401) -> ("error out"=w394:errorcluster, "Data Car Wash Output"=w400:T10)  [unwired: 6 in]
            n101 = call "Timer.vi"("error in (no error)"=w394, "Pause"=w399) -> ("error out"=w393:errorcluster, "Elapsed Time"=w398:dbl)  [unwired: 6 in, 1 out]
          }
          frame 4 {
            w409 = TRUE  # Pause
            # "This case structure checks if the car is at the right station. If it does, continue the sequence of washes; if not, pause the timer and notify the user to drive the car to the right place."
            n102 = call "Cluster Value.vi"("error in (no error)"=w402, "Enum Input"=w405, "Vehicle Out of Position"=TRUE, "Data Car Wash"=w410) -> ("error out"=w404:errorcluster, "Data Car Wash Output"=w411:T10)  [unwired: 6 in]
            n103 = call "Timer.vi"("error in (no error)"=w404, "Pause"=w409) -> ("error out"=w403:errorcluster, "Elapsed Time"=w408:dbl)  [unwired: 6 in, 1 out]
          }
        }
      }
      frame "Low Pressure Wax" {
        # "This case structure controls all the car wash steps, including the startup and shutdown of the program."
        n104 = case shown="2, Default" w415 {
          tunnel: [Enum_State_Machine."Low Pressure Wax" Enum_State_Machine."Low Pressure Wax" w452 Enum_State_Machine."Low Pressure Wax" Enum_State_Machine."Low Pressure Wax"] -> w418
          tunnel: w414 -> [w430 w439 w454 w466 w475]
          tunnel: [w429 w438 w453 w465 w476] -> w413
          tunnel: w416 -> [w425 w434 w445 w460 w470]
          tunnel: [w427 w437 w450 w463 w473] -> w417
          tunnel: [w423 w432 w443 w458 w468] -> w419
          tunnel: w412 -> [w422 _ w442 w457 w467]
          frame 0 {
            w428 = TRUE  # Pause
            # "This case structure checks if the car is at the right station. If it does, continue the sequence of washes; if not, pause the timer and notify the user to drive the car to the right place."
            n105 = call "Cluster Value.vi"("error in (no error)"=w422, "Enum Input"=w425, "Vehicle Out of Position"=TRUE, "Data Car Wash"=w430) -> ("error out"=w424:errorcluster, "Data Car Wash Output"=w429:T10)  [unwired: 6 in]
            n106 = call "Timer.vi"("error in (no error)"=w424, "Pause"=w428) -> ("error out"=w423:errorcluster, "Elapsed Time"=w427:dbl)  [unwired: 6 in, 1 out]
          }
          frame 1 {
            w436 = TRUE  # Pause
            # "This case structure checks if the car is at the right station. If it does, continue the sequence of washes; if not, pause the timer and notify the user to drive the car to the right place."
            n107 = call "Cluster Value.vi"("Enum Input"=w434, "Vehicle Out of Position"=TRUE, "Data Car Wash"=w439) -> ("error out"=w433:errorcluster, "Data Car Wash Output"=w438:T10)  [unwired: 7 in]
            n108 = call "Timer.vi"("error in (no error)"=w433, "Pause"=w436) -> ("error out"=w432:errorcluster, "Elapsed Time"=w437:dbl)  [unwired: 6 in, 1 out]
          }
          frame 2, Default {
            # "If the user doesn't choose this option, it goes directly to the next state. If the user chooses this option, it stays in this case until the time has elapsed."
            # "This case structure checks if the car is at the right station. If it does, continue the sequence of washes; if not, pause the timer and notify the user to drive the car to the right place."
            n109 = call "Cluster Value.vi"("error in (no error)"=w442, "Enum Input"=w445, "Vehicle Out of Position"=FALSE, "Data Car Wash"=w454) -> ("error out"=w444:errorcluster, "Data Car Wash Output"=w453:T10)  [unwired: 6 in]
            n110 = Unbundle By Name(w453) -> ("Wash Options.Low Pressure Wax"=w448:bool)
            n111 = call "Timer.vi"("error in (no error)"=w444, "Pause"=FALSE) -> ("error out"=w443:errorcluster, "Time Has Elapsed?"=w441:bool, "Elapsed Time"=w450:dbl)  [unwired: 6 in]
            n112 = Not(x=w448) -> (.not. x?=w447:bool)
            n113 = Or(x=w447, y=w441) -> (x .or. y?=w449:bool)
            n114 = case shown="True" w449 {
              tunnel: [Enum_State_Machine."Low Pressure Wax" ("Enum") Enum_State_Machine."Spot Free Rinse" ("Enum")] -> w452
              frame False {
              }
              frame True {
              }
            }
          }
          frame 3 {
            w464 = TRUE  # Pause
            # "This case structure checks if the car is at the right station. If it does, continue the sequence of washes; if not, pause the timer and notify the user to drive the car to the right place."
            n115 = call "Cluster Value.vi"("error in (no error)"=w457, "Enum Input"=w460, "Vehicle Out of Position"=TRUE, "Data Car Wash"=w466) -> ("error out"=w459:errorcluster, "Data Car Wash Output"=w465:T10)  [unwired: 6 in]
            n116 = call "Timer.vi"("error in (no error)"=w459, "Pause"=w464) -> ("error out"=w458:errorcluster, "Elapsed Time"=w463:dbl)  [unwired: 6 in, 1 out]
          }
          frame 4 {
            w474 = TRUE  # Pause
            # "This case structure checks if the car is at the right station. If it does, continue the sequence of washes; if not, pause the timer and notify the user to drive the car to the right place."
            n117 = call "Cluster Value.vi"("error in (no error)"=w467, "Enum Input"=w470, "Vehicle Out of Position"=TRUE, "Data Car Wash"=w475) -> ("error out"=w469:errorcluster, "Data Car Wash Output"=w476:T10)  [unwired: 6 in]
            n118 = call "Timer.vi"("error in (no error)"=w469, "Pause"=w474) -> ("error out"=w468:errorcluster, "Elapsed Time"=w473:dbl)  [unwired: 6 in, 1 out]
          }
        }
      }
      frame "Spot Free Rinse" {
        # "This case structure controls all the car wash steps, including the startup and shutdown of the program."
        n119 = case shown="2, Default" w482 {
          tunnel: [Enum_State_Machine."Spot Free Rinse" Enum_State_Machine."Spot Free Rinse" w518 Enum_State_Machine."Spot Free Rinse" Enum_State_Machine."Spot Free Rinse"] -> w479
          tunnel: w483 -> [w495 w505 w520 w532 w541]
          tunnel: [w494 w504 w519 w531 w542] -> w484
          tunnel: w481 -> [w490 w500 w511 w526 w536]
          tunnel: [w492 w503 w516 w529 w539] -> w478
          tunnel: [w488 w498 w509 w524 w534] -> w480
          tunnel: w477 -> [w487 w497 w507 w523 w533]
          frame 0 {
            w493 = TRUE  # Pause
            # "This case structure checks if the car is at the right station. If it does, continue the sequence of washes; if not, pause the timer and notify the user to drive the car to the right place."
            n120 = call "Cluster Value.vi"("error in (no error)"=w487, "Enum Input"=w490, "Vehicle Out of Position"=TRUE, "Data Car Wash"=w495) -> ("error out"=w489:errorcluster, "Data Car Wash Output"=w494:T10)  [unwired: 6 in]
            n121 = call "Timer.vi"("error in (no error)"=w489, "Pause"=w493) -> ("error out"=w488:errorcluster, "Elapsed Time"=w492:dbl)  [unwired: 6 in, 1 out]
          }
          frame 1 {
            w502 = TRUE  # Pause
            # "This case structure checks if the car is at the right station. If it does, continue the sequence of washes; if not, pause the timer and notify the user to drive the car to the right place."
            n122 = call "Cluster Value.vi"("error in (no error)"=w497, "Enum Input"=w500, "Vehicle Out of Position"=TRUE, "Data Car Wash"=w505) -> ("error out"=w499:errorcluster, "Data Car Wash Output"=w504:T10)  [unwired: 6 in]
            n123 = call "Timer.vi"("error in (no error)"=w499, "Pause"=w502) -> ("error out"=w498:errorcluster, "Elapsed Time"=w503:dbl)  [unwired: 6 in, 1 out]
          }
          frame 2, Default {
            # "If the user doesn't choose this option, it goes directly to the next state. If the user chooses this option, it stays in this case until the time has elapsed."
            # "This case structure checks if the car is at the right station. If it does, continue the sequence of washes; if not, pause the timer and notify the user to drive the car to the right place."
            n124 = call "Cluster Value.vi"("error in (no error)"=w507, "Enum Input"=w511, "Vehicle Out of Position"=FALSE, "Data Car Wash"=w520) -> ("error out"=w510:errorcluster, "Data Car Wash Output"=w519:T10)  [unwired: 6 in]
            n125 = Unbundle By Name(w519) -> ("Wash Options.Spot Free Rinse"=w514:bool)
            n126 = call "Timer.vi"("error in (no error)"=w510, "Pause"=FALSE) -> ("error out"=w509:errorcluster, "Time Has Elapsed?"=w508:bool, "Elapsed Time"=w516:dbl)  [unwired: 6 in]
            n127 = Not(x=w514) -> (.not. x?=w513:bool)
            n128 = Or(x=w513, y=w508) -> (x .or. y?=w515:bool)
            n129 = case shown="True" w515 {
              tunnel: [Enum_State_Machine."Spot Free Rinse" ("Enum") Enum_State_Machine."Tire Shine Foam" ("Enum")] -> w518
              frame False {
              }
              frame True {
              }
            }
          }
          frame 3 {
            w530 = TRUE  # Pause
            # "This case structure checks if the car is at the right station. If it does, continue the sequence of washes; if not, pause the timer and notify the user to drive the car to the right place."
            n130 = call "Cluster Value.vi"("error in (no error)"=w523, "Enum Input"=w526, "Vehicle Out of Position"=TRUE, "Data Car Wash"=w532) -> ("error out"=w525:errorcluster, "Data Car Wash Output"=w531:T10)  [unwired: 6 in]
            n131 = call "Timer.vi"("error in (no error)"=w525, "Pause"=w530) -> ("error out"=w524:errorcluster, "Elapsed Time"=w529:dbl)  [unwired: 6 in, 1 out]
          }
          frame 4 {
            w540 = TRUE  # Pause
            # "This case structure checks if the car is at the right station. If it does, continue the sequence of washes; if not, pause the timer and notify the user to drive the car to the right place."
            n132 = call "Cluster Value.vi"("error in (no error)"=w533, "Enum Input"=w536, "Vehicle Out of Position"=TRUE, "Data Car Wash"=w541) -> ("error out"=w535:errorcluster, "Data Car Wash Output"=w542:T10)  [unwired: 6 in]
            n133 = call "Timer.vi"("error in (no error)"=w535, "Pause"=w540) -> ("error out"=w534:errorcluster, "Elapsed Time"=w539:dbl)  [unwired: 6 in, 1 out]
          }
        }
      }
      frame "Tire Shine Foam" {
        # "This case structure controls all the car wash steps, including the startup and shutdown of the program."
        n134 = case shown="3, Default" w548 {
          tunnel: [Enum_State_Machine."Tire Shine Foam" Enum_State_Machine."Tire Shine Foam" Enum_State_Machine."Tire Shine Foam" w594 Enum_State_Machine."Tire Shine Foam"] -> w545
          tunnel: w549 -> [w561 w571 w582 w596 w607]
          tunnel: [w560 w570 w581 w595 w608] -> w550
          tunnel: w547 -> [w556 w566 w576 w587 w602]
          tunnel: [w558 w569 w579 w592 w605] -> w544
          tunnel: [w554 w564 w574 w585 w600] -> w546
          tunnel: w543 -> [w553 w563 w573 w583 w599]
          frame 0 {
            w559 = TRUE  # Pause
            # "This case structure checks if the car is at the right station. If it does, continue the sequence of washes; if not, pause the timer and notify the user to drive the car to the right place."
            n135 = call "Cluster Value.vi"("error in (no error)"=w553, "Enum Input"=w556, "Vehicle Out of Position"=TRUE, "Data Car Wash"=w561) -> ("error out"=w555:errorcluster, "Data Car Wash Output"=w560:T10)  [unwired: 6 in]
            n136 = call "Timer.vi"("error in (no error)"=w555, "Pause"=w559) -> ("error out"=w554:errorcluster, "Elapsed Time"=w558:dbl)  [unwired: 6 in, 1 out]
          }
          frame 1 {
            w568 = TRUE  # Pause
            # "This case structure checks if the car is at the right station. If it does, continue the sequence of washes; if not, pause the timer and notify the user to drive the car to the right place."
            n137 = call "Cluster Value.vi"("error in (no error)"=w563, "Enum Input"=w566, "Vehicle Out of Position"=TRUE, "Data Car Wash"=w571) -> ("error out"=w565:errorcluster, "Data Car Wash Output"=w570:T10)  [unwired: 6 in]
            n138 = call "Timer.vi"("error in (no error)"=w565, "Pause"=w568) -> ("error out"=w564:errorcluster, "Elapsed Time"=w569:dbl)  [unwired: 6 in, 1 out]
          }
          frame 2 {
            w580 = TRUE  # Pause
            # "This case structure checks if the car is at the right station. If it does, continue the sequence of washes; if not, pause the timer and notify the user to drive the car to the right place."
            n139 = call "Cluster Value.vi"("error in (no error)"=w573, "Enum Input"=w576, "Vehicle Out of Position"=TRUE, "Data Car Wash"=w582) -> ("error out"=w575:errorcluster, "Data Car Wash Output"=w581:T10)  [unwired: 6 in]
            n140 = call "Timer.vi"("error in (no error)"=w575, "Pause"=w580) -> ("error out"=w574:errorcluster, "Elapsed Time"=w579:dbl)  [unwired: 6 in, 1 out]
          }
          frame 3, Default {
            # "If the user doesn't choose this option, it goes directly to the next state. If the user chooses this option, it stays in this case until the time has elapsed."
            # "This case structure checks if the car is at the right station. If it does, continue the sequence of washes; if not, pause the timer and notify the user to drive the car to the right place."
            n141 = call "Cluster Value.vi"("error in (no error)"=w583, "Enum Input"=w587, "Vehicle Out of Position"=FALSE, "Data Car Wash"=w596) -> ("error out"=w586:errorcluster, "Data Car Wash Output"=w595:T10)  [unwired: 6 in]
            n142 = Unbundle By Name(w595) -> ("Wash Options.Tire Shine Foam"=w590:bool)
            n143 = call "Timer.vi"("error in (no error)"=w586, "Pause"=FALSE) -> ("error out"=w585:errorcluster, "Time Has Elapsed?"=w584:bool, "Elapsed Time"=w592:dbl)  [unwired: 6 in]
            n144 = Not(x=w590) -> (.not. x?=w589:bool)
            n145 = Or(x=w589, y=w584) -> (x .or. y?=w591:bool)
            n146 = case shown="True" w591 {
              tunnel: [Enum_State_Machine."Tire Shine Foam" ("Enum") Enum_State_Machine."Air Dry" ("Enum")] -> w594
              frame False {
              }
              frame True {
              }
            }
          }
          frame 4 {
            w606 = TRUE  # Pause
            # "This case structure checks if the car is at the right station. If it does, continue the sequence of washes; if not, pause the timer and notify the user to drive the car to the right place."
            n147 = call "Cluster Value.vi"("error in (no error)"=w599, "Enum Input"=w602, "Vehicle Out of Position"=TRUE, "Data Car Wash"=w607) -> ("error out"=w601:errorcluster, "Data Car Wash Output"=w608:T10)  [unwired: 6 in]
            n148 = call "Timer.vi"("error in (no error)"=w601, "Pause"=w606) -> ("error out"=w600:errorcluster, "Elapsed Time"=w605:dbl)  [unwired: 6 in, 1 out]
          }
        }
      }
      frame "Air Dry" {
        # "This case structure controls all the car wash steps, including the startup and shutdown of the program."
        n149 = case shown="3, Default" w614 {
          tunnel: [Enum_State_Machine."Air Dry" Enum_State_Machine."Air Dry" Enum_State_Machine."Air Dry" w660 Enum_State_Machine."Air Dry"] -> w610
          tunnel: w616 -> [w627 w637 w648 w662 w673]
          tunnel: [w626 w636 w647 w661 w674] -> w615
          tunnel: w613 -> [w622 w632 w642 w653 w668]
          tunnel: [w624 w635 w645 w658 w671] -> w611
          tunnel: [w620 w630 w640 w651 w666] -> w612
          tunnel: w609 -> [w619 w629 w639 w649 w665]
          frame 0 {
            w625 = TRUE  # Pause
            # "This case structure checks if the car is at the right station. If it does, continue the sequence of washes; if not, pause the timer and notify the user to drive the car to the right place."
            n150 = call "Cluster Value.vi"("error in (no error)"=w619, "Enum Input"=w622, "Vehicle Out of Position"=TRUE, "Data Car Wash"=w627) -> ("error out"=w621:errorcluster, "Data Car Wash Output"=w626:T10)  [unwired: 6 in]
            n151 = call "Timer.vi"("error in (no error)"=w621, "Pause"=w625) -> ("error out"=w620:errorcluster, "Elapsed Time"=w624:dbl)  [unwired: 6 in, 1 out]
          }
          frame 1 {
            w634 = TRUE  # Pause
            # "This case structure checks if the car is at the right station. If it does, continue the sequence of washes; if not, pause the timer and notify the user to drive the car to the right place."
            n152 = call "Cluster Value.vi"("error in (no error)"=w629, "Enum Input"=w632, "Vehicle Out of Position"=TRUE, "Data Car Wash"=w637) -> ("error out"=w631:errorcluster, "Data Car Wash Output"=w636:T10)  [unwired: 6 in]
            n153 = call "Timer.vi"("error in (no error)"=w631, "Pause"=w634) -> ("error out"=w630:errorcluster, "Elapsed Time"=w635:dbl)  [unwired: 6 in, 1 out]
          }
          frame 2 {
            w646 = TRUE  # Pause
            # "This case structure checks if the car is at the right station. If it does, continue the sequence of washes; if not, pause the timer and notify the user to drive the car to the right place."
            n154 = call "Cluster Value.vi"("error in (no error)"=w639, "Enum Input"=w642, "Vehicle Out of Position"=TRUE, "Data Car Wash"=w648) -> ("error out"=w641:errorcluster, "Data Car Wash Output"=w647:T10)  [unwired: 6 in]
            n155 = call "Timer.vi"("error in (no error)"=w641, "Pause"=w646) -> ("error out"=w640:errorcluster, "Elapsed Time"=w645:dbl)  [unwired: 6 in, 1 out]
          }
          frame 3, Default {
            # "If the user doesn't choose this option, it goes directly to the next state. If the user chooses this option, it stays in this case until the time has elapsed."
            # "This case structure checks if the car is at the right station. If it does, continue the sequence of washes; if not, pause the timer and notify the user to drive the car to the right place."
            n156 = call "Cluster Value.vi"("error in (no error)"=w649, "Enum Input"=w653, "Vehicle Out of Position"=FALSE, "Data Car Wash"=w662) -> ("error out"=w652:errorcluster, "Data Car Wash Output"=w661:T10)  [unwired: 6 in]
            n157 = Unbundle By Name(w661) -> ("Wash Options.Air Dry"=w656:bool)
            n158 = call "Timer.vi"("error in (no error)"=w652, "Pause"=FALSE) -> ("error out"=w651:errorcluster, "Time Has Elapsed?"=w650:bool, "Elapsed Time"=w658:dbl)  [unwired: 6 in]
            n159 = Not(x=w656) -> (.not. x?=w655:bool)
            n160 = Or(x=w655, y=w650) -> (x .or. y?=w657:bool)
            n161 = case shown="True" w657 {
              tunnel: [Enum_State_Machine."Air Dry" ("Enum") Enum_State_Machine."Exit" ("Enum")] -> w660
              frame False {
              }
              frame True {
              }
            }
          }
          frame 4 {
            w672 = TRUE  # Pause
            # "This case structure checks if the car is at the right station. If it does, continue the sequence of washes; if not, pause the timer and notify the user to drive the car to the right place."
            n162 = call "Cluster Value.vi"("error in (no error)"=w665, "Enum Input"=w668, "Vehicle Out of Position"=TRUE, "Data Car Wash"=w673) -> ("error out"=w667:errorcluster, "Data Car Wash Output"=w674:T10)  [unwired: 6 in]
            n163 = call "Timer.vi"("error in (no error)"=w667, "Pause"=w672) -> ("error out"=w666:errorcluster, "Elapsed Time"=w671:dbl)  [unwired: 6 in, 1 out]
          }
        }
      }
      frame "Exit" {
        # "This case structure controls all the car wash steps, including the startup and shutdown of the program."
        n164 = case shown="4, Default" w679 {
          tunnel: [Enum_State_Machine."Exit" Enum_State_Machine."Exit" Enum_State_Machine."Exit" Enum_State_Machine."Exit" Enum_State_Machine."Startup"] -> w680
          tunnel: w683 -> [w690 w696 w704 w711 w718]
          tunnel: [w689 w697 w703 w710 w719] -> w682
          tunnel: w681 -> [w687 w694 w701 w708 w715]
          tunnel: [w686 w693 w700 w707 w714] -> w676
          tunnel: w675 -> [w685 w692 w699 w706 w713]
          frame 0 {
            # "This case structure checks if the car is at the right station. If it does, continue the sequence of washes; if not, pause the timer and notify the user to drive the car to the right place."
            n165 = call "Cluster Value.vi"("error in (no error)"=w685, "Enum Input"=w687, "Vehicle Out of Position"=TRUE, "Data Car Wash"=w690) -> ("error out"=w686:errorcluster, "Data Car Wash Output"=w689:T10)  [unwired: 6 in]
          }
          frame 1 {
            # "This case structure checks if the car is at the right station. If it does, continue the sequence of washes; if not, pause the timer and notify the user to drive the car to the right place."
            n166 = call "Cluster Value.vi"("error in (no error)"=w692, "Enum Input"=w694, "Vehicle Out of Position"=TRUE, "Data Car Wash"=w696) -> ("error out"=w693:errorcluster, "Data Car Wash Output"=w697:T10)  [unwired: 6 in]
          }
          frame 2 {
            # "This case structure checks if the car is at the right station. If it does, continue the sequence of washes; if not, pause the timer and notify the user to drive the car to the right place."
            n167 = call "Cluster Value.vi"("error in (no error)"=w699, "Enum Input"=w701, "Vehicle Out of Position"=TRUE, "Data Car Wash"=w704) -> ("error out"=w700:errorcluster, "Data Car Wash Output"=w703:T10)  [unwired: 6 in]
          }
          frame 3 {
            # "This case structure checks if the car is at the right station. If it does, continue the sequence of washes; if not, pause the timer and notify the user to drive the car to the right place."
            n168 = call "Cluster Value.vi"("error in (no error)"=w706, "Enum Input"=w708, "Vehicle Out of Position"=TRUE, "Data Car Wash"=w711) -> ("error out"=w707:errorcluster, "Data Car Wash Output"=w710:T10)  [unwired: 6 in]
          }
          frame 4, Default {
            # "Restart the program"
            # "This case structure checks if the car is at the right station. If it does, continue the sequence of washes; if not, pause the timer and notify the user to drive the car to the right place."
            n169 = call "Cluster Value.vi"("error in (no error)"=w713, "Enum Input"=w715, "Vehicle Out of Position"=FALSE, "Data Car Wash"=w718) -> ("error out"=w714:errorcluster, "Data Car Wash Output"=w719:T10)  [unwired: 6 in]
          }
        }
      }
      frame "Stop" {
        w729 = TRUE  # Reset
        w732 = FALSE  # Vehicle Out of Position
        # "This case structure controls all the car wash steps, including the startup and shutdown of the program."
        n170 = control-ref of="Water Flow Graph"() -> (w720:refnum<vi>)
        n171 = control-ref of="Start"() -> (w723:refnum<vi>)
        n172 = control-ref of="Wash Options"() -> (w725:refnum<vi>)
        n173 = control-ref of="Car Position Slider"() -> (w724:refnum<vi>)
        n174 = control-ref of="Duty Cycle Control(%)"() -> (w722:refnum<vi>)
        n175 = call "Set Front Panel Properties.vi"("Water Flow Graph Refnum"=w720, "Wash Op Refnum"=w725, "Car Slider Refnum"=w724, "error in (no error)"=w726, "Control"=T9."Enabled", "DtCy Slider Refnum"=w722, "Start Refnum"=w723) -> ("error out"=w727:errorcluster)  [unwired: 4 in]
        n176 = call "Cluster Value.vi"("error in (no error)"=w727, "Enum Input"=w731, "Vehicle Out of Position"=w732, "Data Car Wash"=w736) -> ("error out"=w728:errorcluster, "Data Car Wash Output"=w735:T10)  [unwired: 6 in]
        n177 = call "Timer.vi"("error in (no error)"=w728, "Reset"=w729) -> ("error out"=w730:errorcluster)  [unwired: 6 in, 2 out]
      }
    }
    "Wash Entry" <- w96
    "Elapsed Time" <- w95
    n178 = Unbundle By Name(w93) -> ("Car Wash Indicators"=w90:T2)
    "CW Indicators" <- w90
    n179 = call "Digital Output Control VI.vi"("Car Wash Indicators"=w90) -> ()  [unwired: 11 in]
  }
  n180 = Merge Errors(w8, w18) -> (w11:errorcluster)
  n181 = Release Queue(queue=w9, error in (no error)=w11) -> (error out=w10:errorcluster)  [unwired: 1 in, 2 out]
  n182 = call <vilib>:"Simple Error Handler.vi"("error in (no error)"=w10) -> ("error out"=→"error out":errorcluster)  [unwired: 4 in, 4 out]
